vi "Init Active Devices.vi"(8 "error in":errorcluster, 10 "Device Names":string, 11 "DAC HeatFlow AIV in":refnum<class "DAC HeatFlow AOV.lvclass">) -> (0 "error out":errorcluster, 3 "DAC HeatFlow AIV out":refnum<class "DAC HeatFlow AOV.lvclass">)   [LabVIEW 2019, in "DAC.lvlib" / "DAC HeatFlow AOV.lvclass"]
uses:
  DAC HeatFlow AOV.lvclass
  DAC HeatFlow AOV.lvclass/DAC HeatFlow AOV.ctl
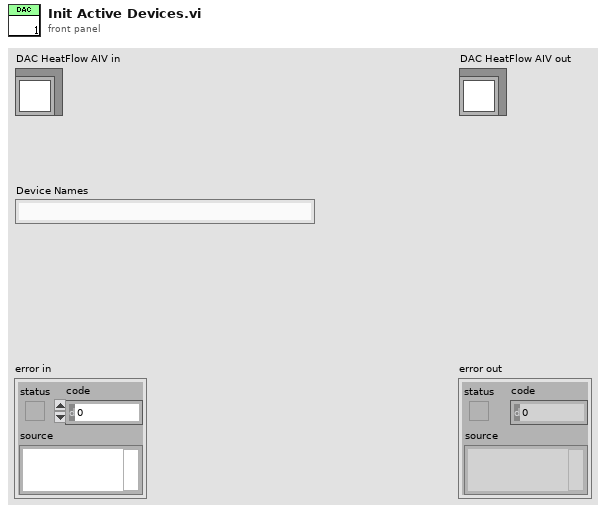
[diagram p1: front panel]
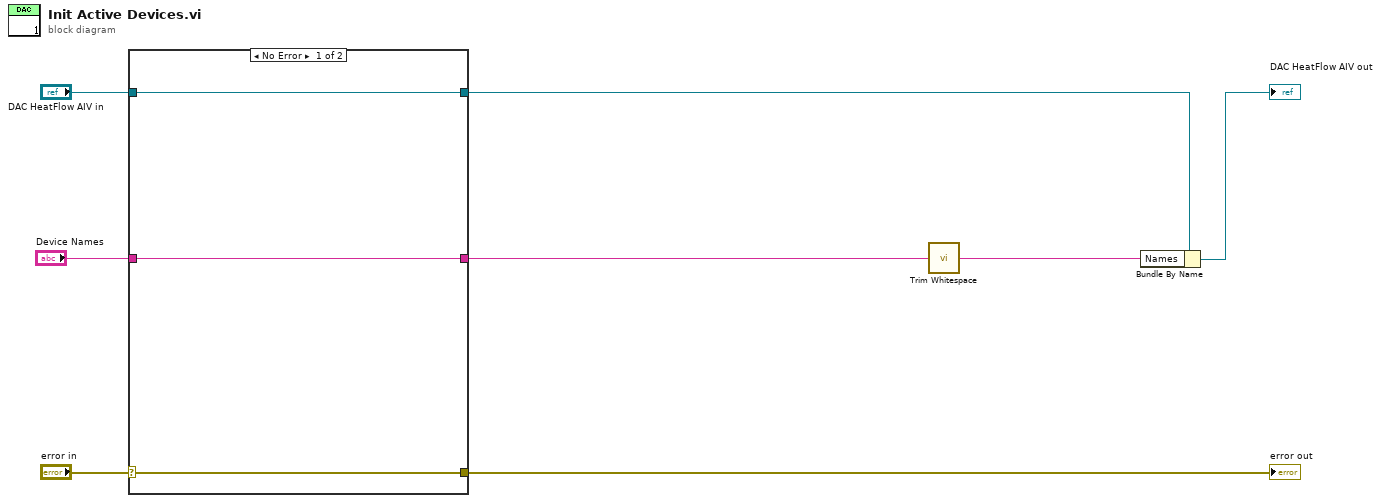
[diagram p0: block diagram]
diagram:
  n1 = case shown="No Error" "error in" {
    selector: "error in" -> [w11 w14]
    tunnel: [w11 w14] -> w7
    tunnel: [w10 w13] -> w5
    tunnel: "DAC HeatFlow AIV in" -> [w10 w13]
    tunnel: "Device Names" -> [w9 w12]
    tunnel: [w9 w12] -> w2
    frame No Error {
    }
    frame Error {
    }
  }
  "error out" <- w7
  n2 = call <vilib>:"Trim Whitespace.vi"("string"=w2) -> ("trimmed string"=w1:string)  [unwired: 1 in]
  n3 = Bundle By Name(cluster=w5, "Names"=w1) -> (→"DAC HeatFlow AIV out":refnum<class "DAC HeatFlow AOV.lvclass">)
